vi "Ouput_pulse_train.vi"(8 "error in (no error)":errorcluster, 11 "Combine_pulses in":refnum<class "Combine_pulses.lvclass">) -> (0 "error out":errorcluster, 3 "Combine_pulses out":refnum<class "Combine_pulses.lvclass">)   [LabVIEW 2019, in "Combine_pulses.lvclass"]
uses:
  Combine_pulses.lvclass
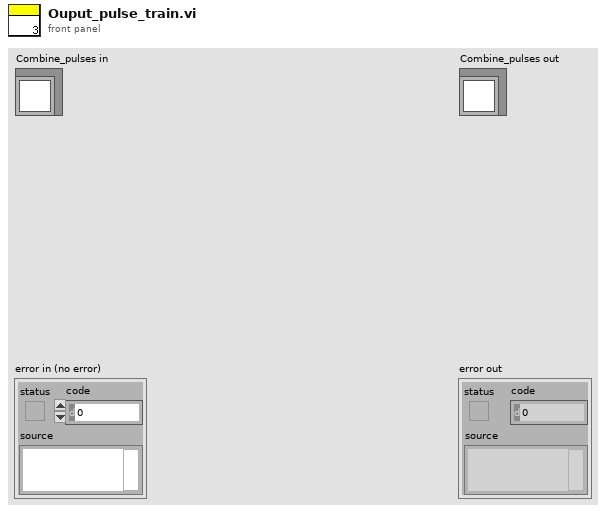
[diagram p1: front panel]
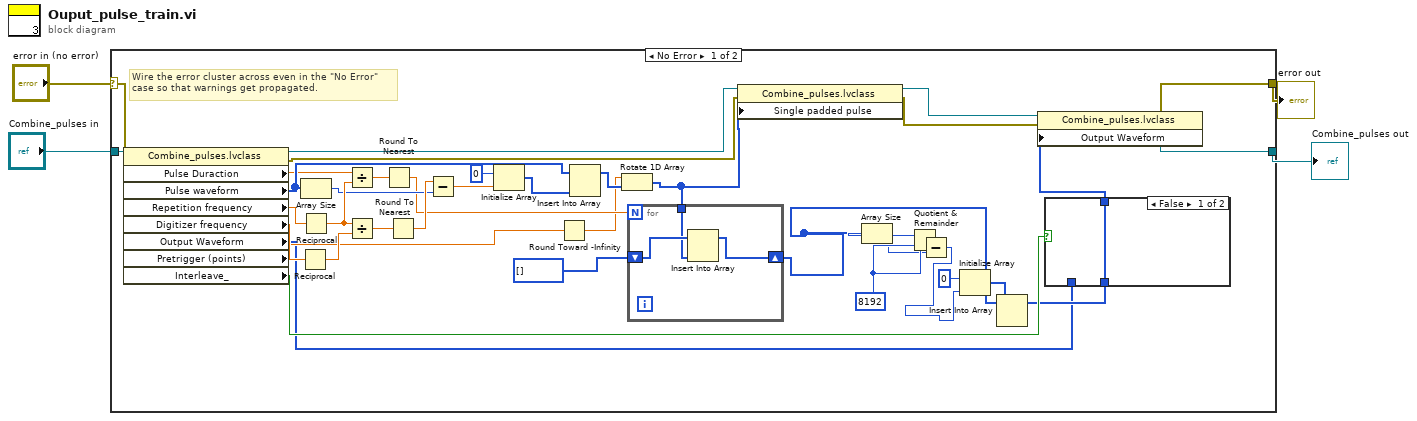
[diagram p0: block diagram]
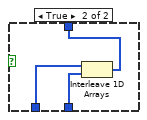
[diagram p2: hidden frame]
diagram:
  n1 = case shown="No Error" "error in (no error)" {
    selector: "error in (no error)" -> [w28 w51]
    tunnel: [w26 w51] -> w3
    tunnel: [w27 w50] -> w1
    tunnel: "Combine_pulses in" -> [w42 w50]
    frame No Error {
      w24 = 8192
      # "Wire the error cluster across even in the \"No Error\"\ncase so that warnings get propagated."
      n2 = property class="Combine_pulses.lvclass"(reference=w42, error in=w28) -> (reference out=w20:refnum<class "Combine_pulses.lvclass">, error out=w18:errorcluster, "Pulse Duraction"=w5:dbl, "Pulse waveform"=w32:i8[], "Repetition frequency"=w41:dbl, "Digitizer frequency"=w39:dbl, "Output Waveform"=w6:i8[], "Pretrigger (points)"=w12:dbl, "Interleave_"=w9:bool)
      n3 = Reciprocal(x=w39) -> (1/x=w30:dbl)
      n4 = Array Size(array=w32) -> (size(s)=w35:i32)
      n5 = Reciprocal(x=w41) -> (1/x=w38:dbl)
      n6 = Divide(x=w5, y=w38) -> (x/y=w40:dbl)
      n7 = Divide(x=w38, y=w30) -> (x/y=w37:dbl)
      n8 = Round To Nearest(number=w40) -> (nearest integer value=w29:dbl)
      n9 = Round To Nearest(number=w37) -> (nearest integer value=w36:dbl)
      n10 = Subtract(x=w36, y=w35) -> (x-y=w33:dbl)
      n11 = Initialize Array(i16 0 ("element"), w33) -> (w31:i16[])
      n12 = Round Toward -Infinity(1:w12) -> (0:w11:dbl)
      n13 = Insert Into Array(array=w32, new element=w31) -> (w14:i8[])  [unwired: 1 in]
      n14 = Rotate 1D Array(1:w14, 2:w11) -> (0:w13:i8[])
      n15 = for {
        N: w29 -> [_]
        shift-right: [w47] -> w15
        shift-left: i8[] [] -> [w49]
        tunnel: w13 -> [w48]
        n16 = Insert Into Array(array=w49, new element=w48) -> (w47:i8[])  [unwired: 1 in]
      }
      n17 = property class="Combine_pulses.lvclass"(reference=w20, error in=w18, "Single padded pulse"=w13) -> (reference out=w19:refnum<class "Combine_pulses.lvclass">, error out=w17:errorcluster)
      n18 = Array Size(array=w15) -> (size(s)=w25:i32)
      n19 = Quotient & Remainder(x=w25, y=w24) -> (x-y*floor(x/y)=w23:i32)  [unwired: 1 out]
      n20 = Subtract(x=w24, y=w23) -> (x-y=w16:i32)
      n21 = Initialize Array(i16 0 ("element"), w16) -> (w21:i16[])
      n22 = Insert Into Array(array=w15, new element=w21) -> (w8:i8[])  [unwired: 1 in]
      n23 = case shown="False" w9 {
        tunnel: w8 -> [w43 w45]
        tunnel: [w43 w44] -> w7
        tunnel: w6 -> [_ w46]
        frame False {
        }
        frame True {
          n24 = Interleave 1D Arrays(w46, w45) -> (w44:i8[])
        }
      }
      n25 = property class="Combine_pulses.lvclass"(reference=w19, error in=w17, "Output Waveform"=w7) -> (reference out=w27:refnum<class "Combine_pulses.lvclass">, error out=w26:errorcluster)
    }
    frame Error {
    }
  }
  "error out" <- w3
  "Combine_pulses out" <- w1
